vi "Auto Inspection_Status.vi"(2 "Action":enum16{"Initial", "Write", "Read"}(ring)=enum."Read", 5 "DataIn":string, 7 "Station":T2, 9 "Data":T1, 11 "error in":errorcluster) -> (4 "Table Control":string[][](table), 6 "DataOut":string, 15 "error out":errorcluster)   [LabVIEW 2019]
uses:
  Ctrl/Auto Inspection Station Name2.ctl
  Ctrl/Auto Inspection Data Name.ctl
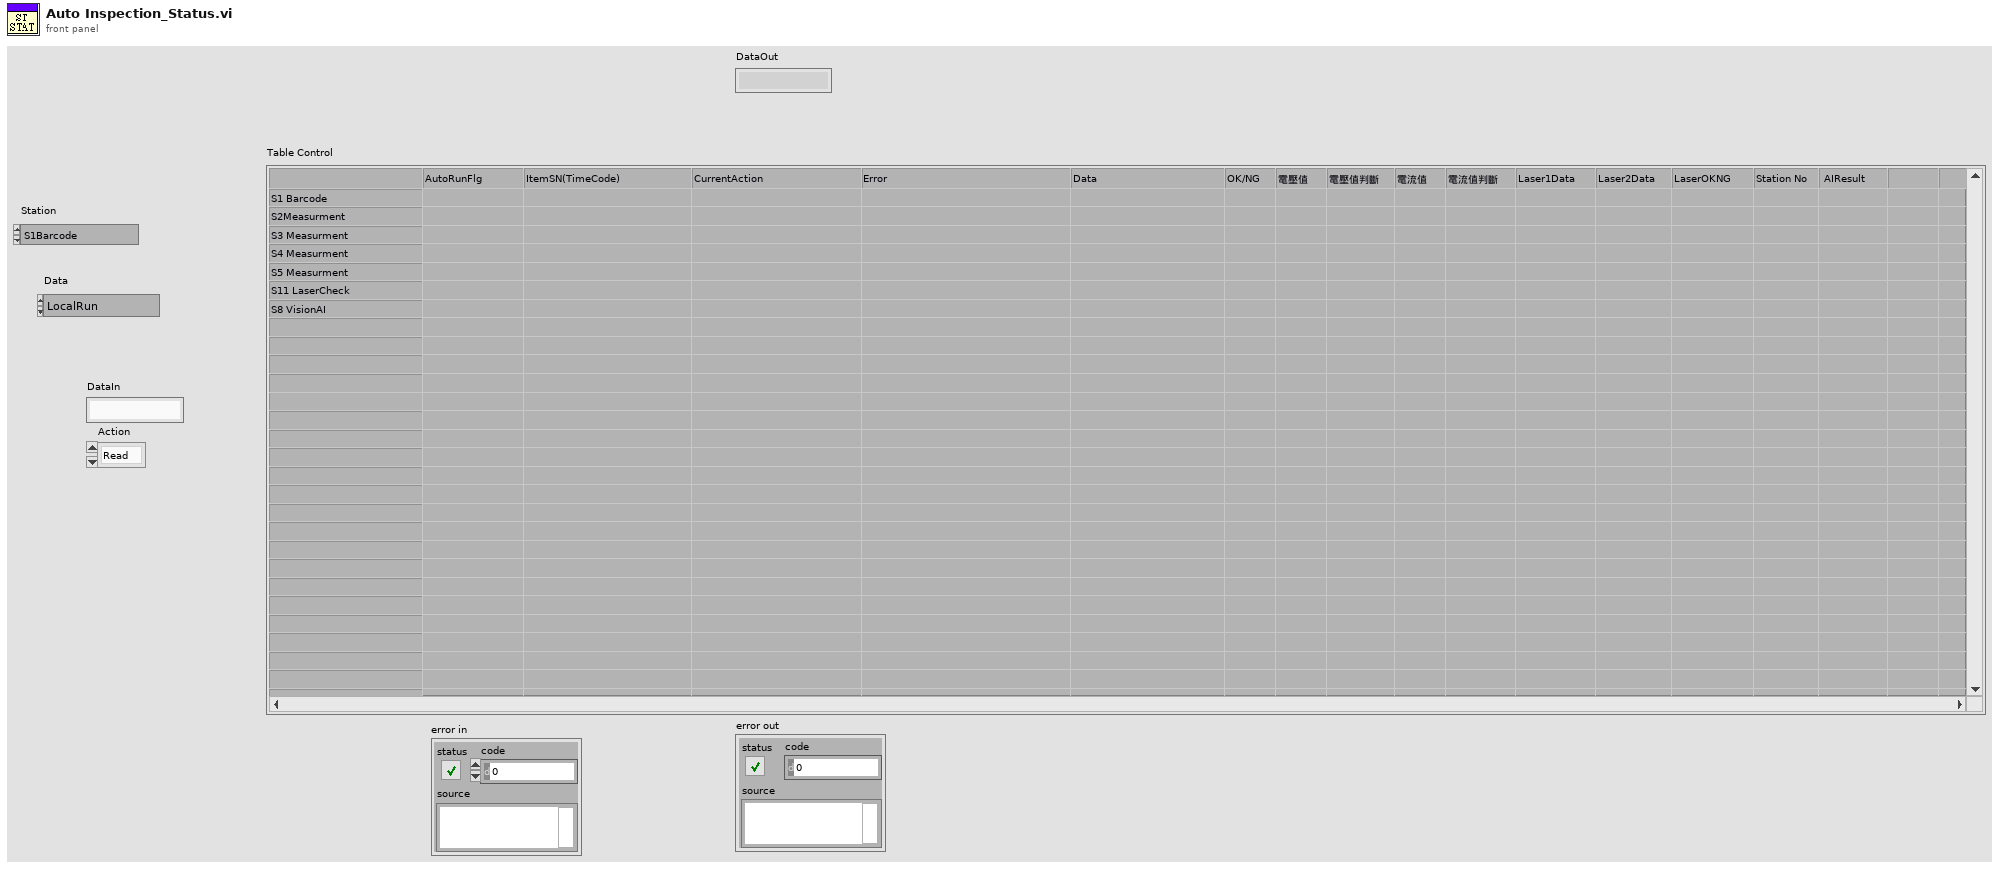
[diagram p1: front panel]
types:
  T1 = typedef "Auto Inspection Data Name.ctl" = enum16{"LocalRun", "ItemSN(TimeCode)", "CurrentAction", "Error", "Data", "OKNG", "電壓值", "電壓值判斷", "電流值", "電流值判斷", "Laser1 Data", "Laser2 Data", "Laser OKNG", "StationNO"}
  T2 = typedef "Auto Inspection Station Name2.ctl" = enum16{"S1Barcode", "S2Measure", "S3Measure", "S4Measure", "S5Measure", "S11_LaserCheck", "S8_Vision AI"}
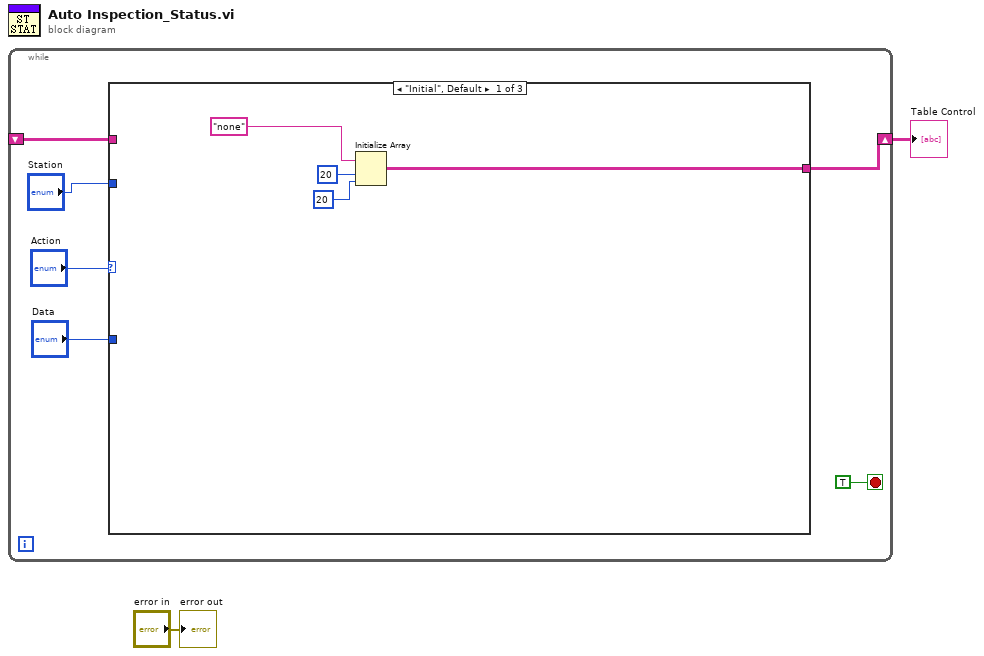
[diagram p0: block diagram]
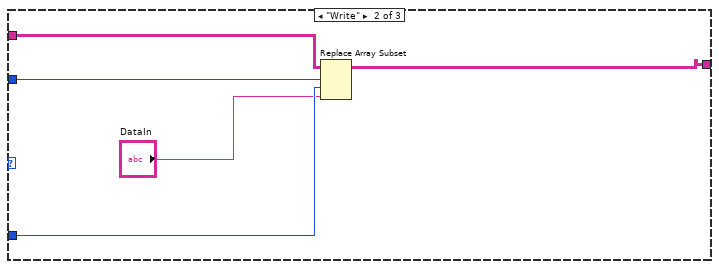
[diagram p2: hidden frame]
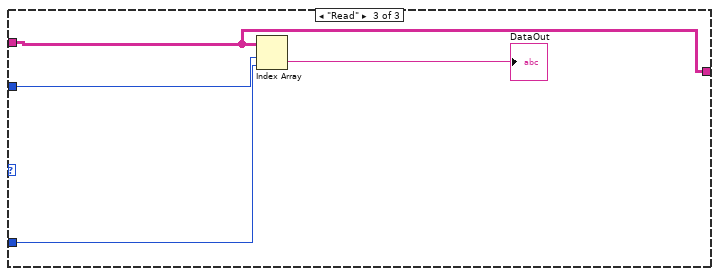
[diagram p3: hidden frame]
diagram:
  n1 = while {
    shift-right: [w7] -> w1
    shift-left: _ -> [w5]
    stop <- TRUE stop-if-true
    n2 = case shown="\"Initial\", Default" "Action" {
      tunnel: [w9 w16 w18] -> w7
      tunnel: w5 -> [_ w17 w18]
      tunnel: "Station" -> [_ w15 w21]
      tunnel: "Data" -> [_ w14 w20]
      frame "Initial", Default {
        n3 = Initialize Array("none", 20 ("dimension size"), 20 ("dimension size")) -> (w9:string[][])
      }
      frame "Write" {
        n4 = Replace Array Subset(array=w17, new element="DataIn", index (row)=w15, index (col)=w14) -> (w16:string[][])
      }
      frame "Read" {
        n5 = Index Array(array=w18, index (row)=w21, index (col)=w20) -> (element=→"DataOut":string)
      }
    }
  }
  "Table Control" <- w1
  "error out" <- "error in"
